vi "test - TMO of Sync-Reply.vi"(8 "error in (no error)":errorcluster, 11 "TestCase in":refnum<class "testcase-Basic-Function.lvclass">) -> (0 "error out":errorcluster, 3 "TestCase out":refnum<class "testcase-Basic-Function.lvclass">)   [LabVIEW 2017, in "testcase-Basic-Function.lvclass"]
uses:
  testcase-Basic-Function.lvclass
  src/user.lib/_NEVSTOP/Communicable State Machine(CSM)/AdvanceAPI/CSM - Revert Arguments-Safe String.vi
  src/user.lib/_NEVSTOP/Communicable State Machine(CSM)/_Shared/Trim Single-line Text.vi
  src/user.lib/_NEVSTOP/Communicable State Machine(CSM)/AdvanceAPI/CSM - Make String Arguments Safe.vi
  src/user.lib/_NEVSTOP/Communicable State Machine(CSM)/AdvanceAPI/CSM - Break Down Multiple States String.vi
  src/user.lib/_NEVSTOP/Communicable State Machine(CSM)/AdvanceAPI/CSM - Compact Multiple States.vi
  src/user.lib/_NEVSTOP/Communicable State Machine(CSM)/AdvanceAPI/CSM - Keywords.vi
  <vilib>/addons/_JKI Toolkits/VI Tester/TestCase.llb/TestCase.lvclass
  src/user.lib/_NEVSTOP/Communicable State Machine(CSM)/Communicable State Machine.lvlib
  C:/Program Files (x86)/National Instruments/LabVIEW 2017/vi.lib/addons/_JKI Toolkits/VI Tester/TestCase.llb/TestCase.lvclass
panel:
  out "x-y":u32
  out "State History":string
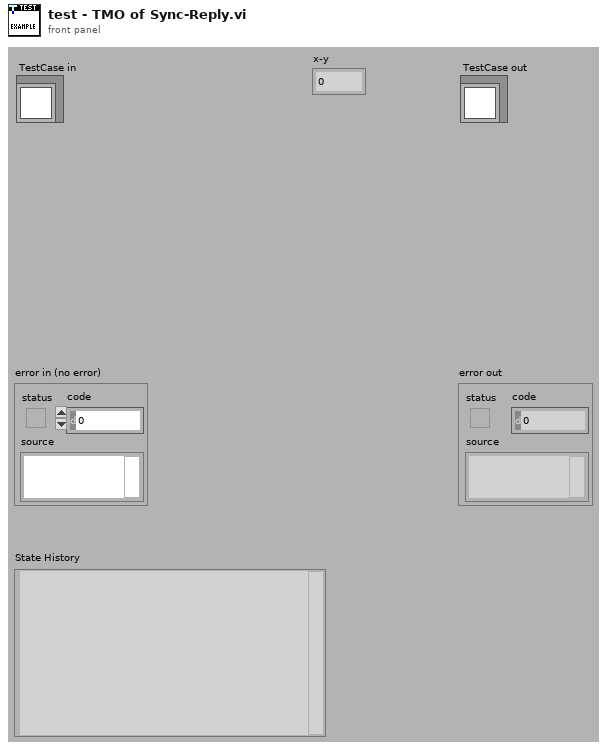
[diagram p1: front panel]
types:
  T1 = enum32{"Invalid", "Standard", "Closed", "Hidden", "Minimized", "Maximized"}
  T2 = enum32{"invalid app kind", "Development System", "Run Time System", "Student Edition", "Embedded LabVIEW", "Evaluation", "Custom"}
  T3 = typedef "Communicable State Machine.lvlib/_CSM_Response Source Message.ctl" = cluster{"‘State":string, "’Arguments":string, "’Error":errorcluster}
  T4 = cluster{"Current VI Reference":refnum<vi>, "Close Panel on Exit?":bool}
  T5 = cluster{"Core":cluster{"Current VI Reference":refnum<vi>, "Close Panel on Exit?":bool}, "Your Boolean data":bool, "Your string data":string}
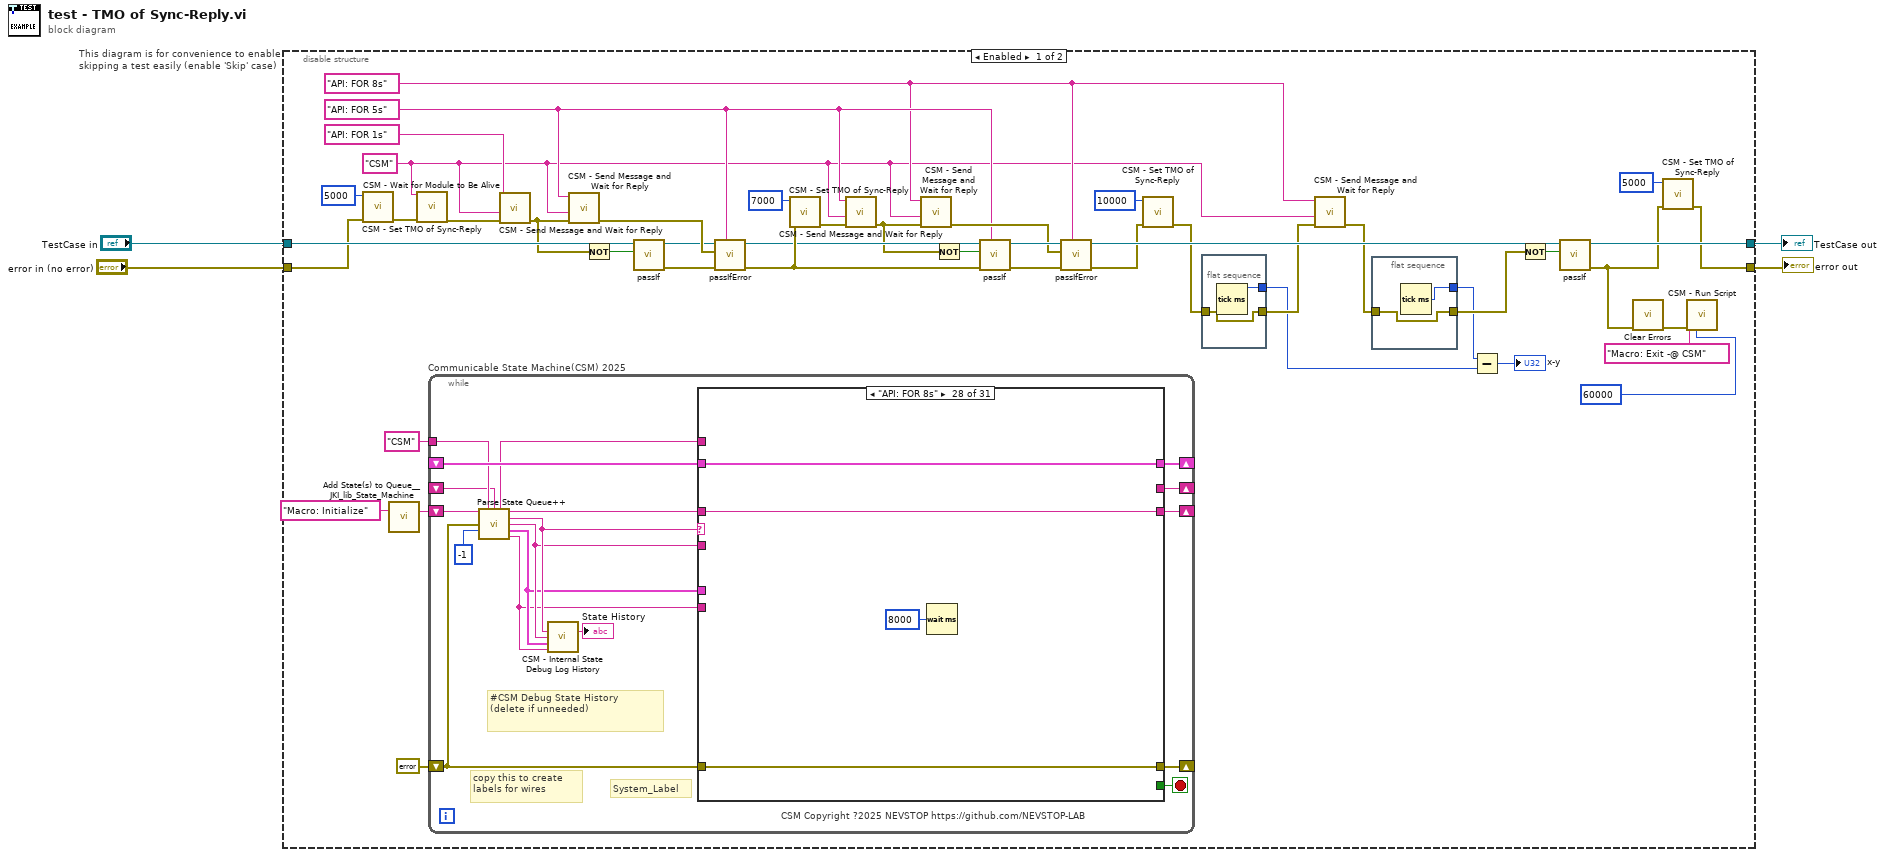
[diagram p0: block diagram]
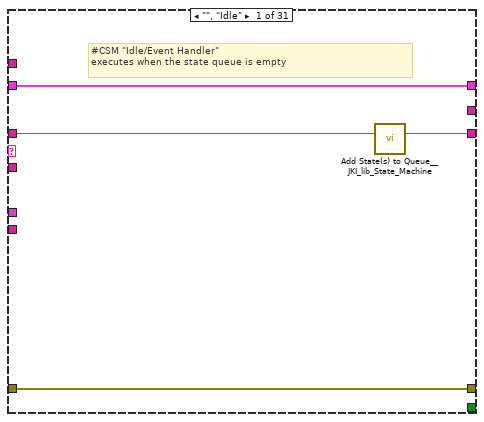
[diagram p2: hidden frame]
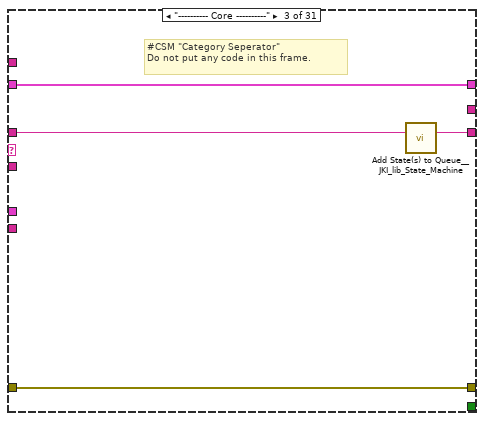
[diagram p4: hidden frame]
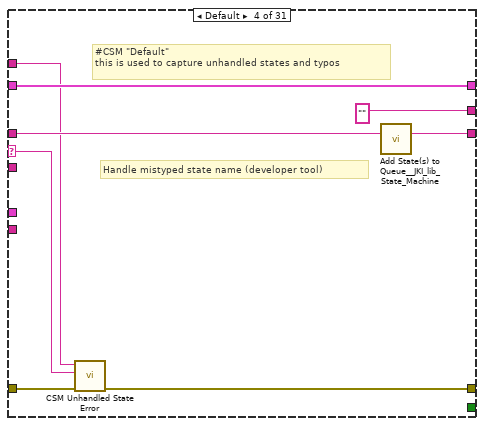
[diagram p5: hidden frame]
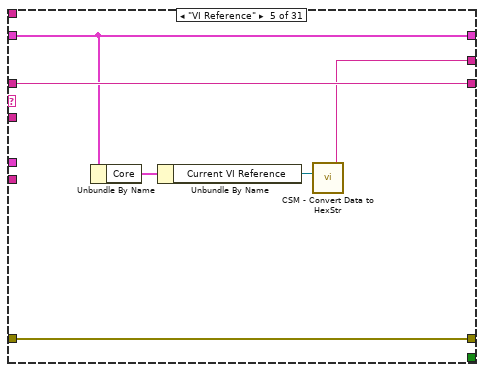
[diagram p6: hidden frame]
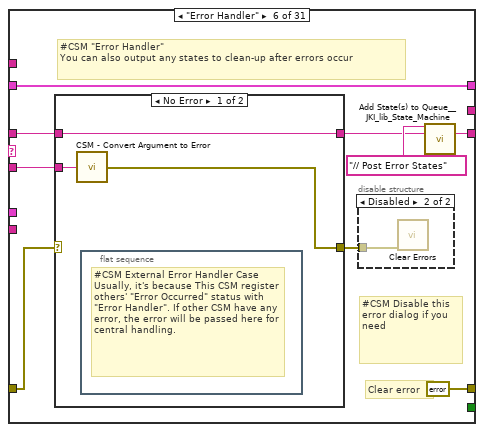
[diagram p7: hidden frame]
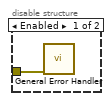
[diagram p8: hidden frame]
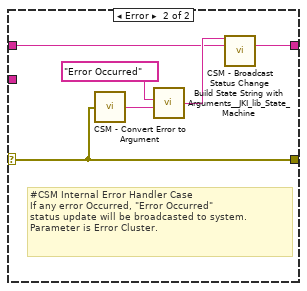
[diagram p9: hidden frame]
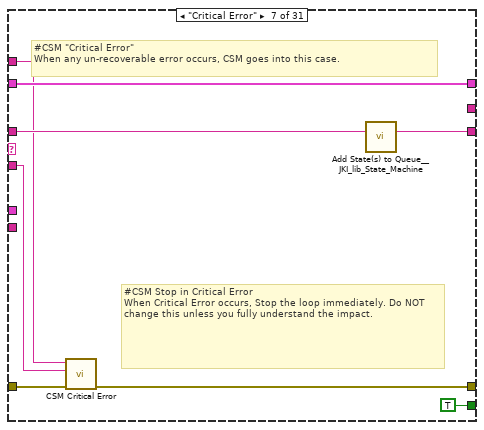
[diagram p10: hidden frame]
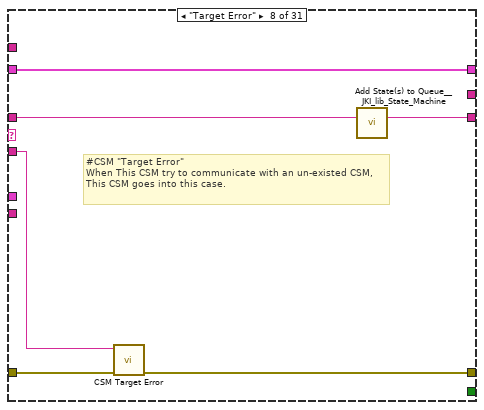
[diagram p11: hidden frame]
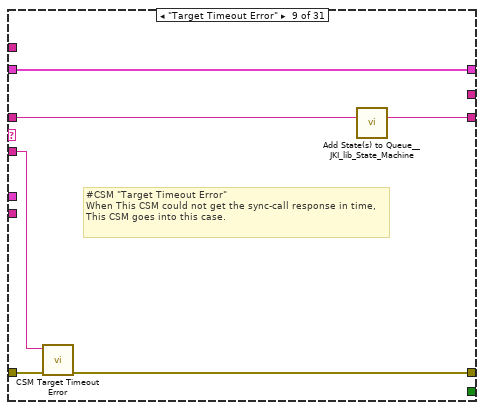
[diagram p12: hidden frame]
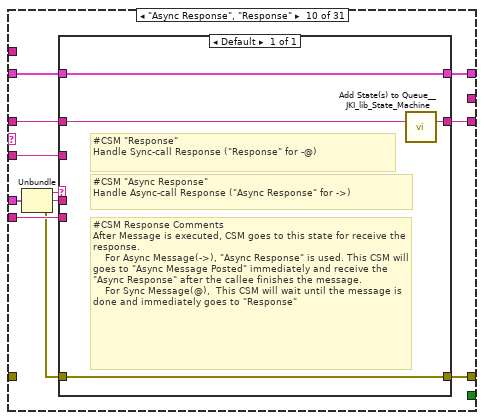
[diagram p13: hidden frame]
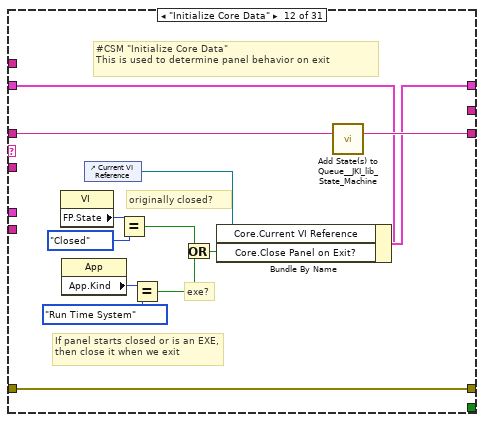
[diagram p15: hidden frame]
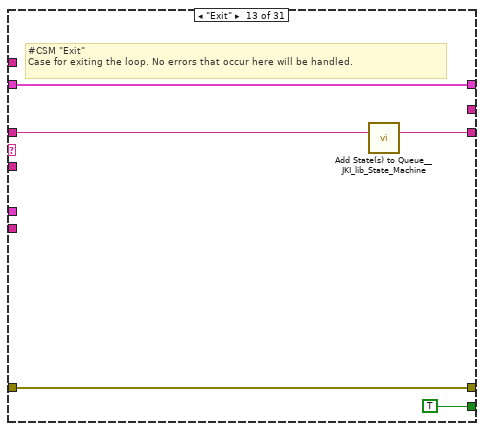
[diagram p16: hidden frame]
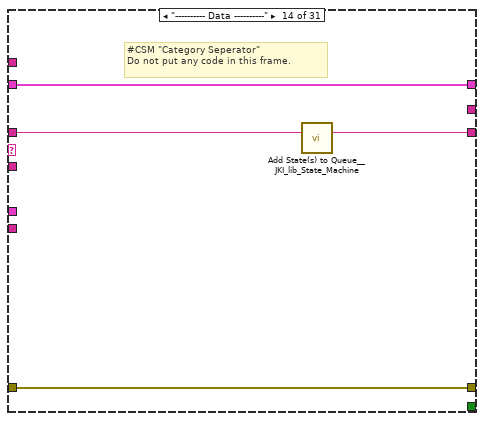
[diagram p17: hidden frame]
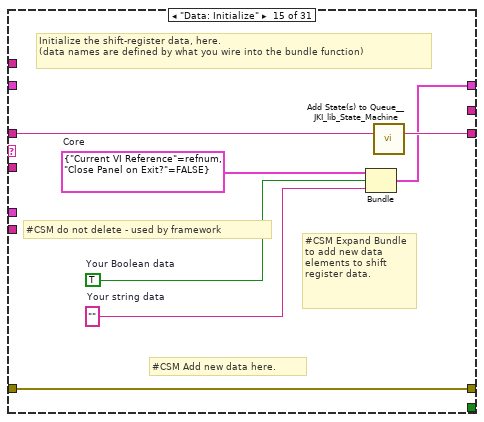
[diagram p18: hidden frame]
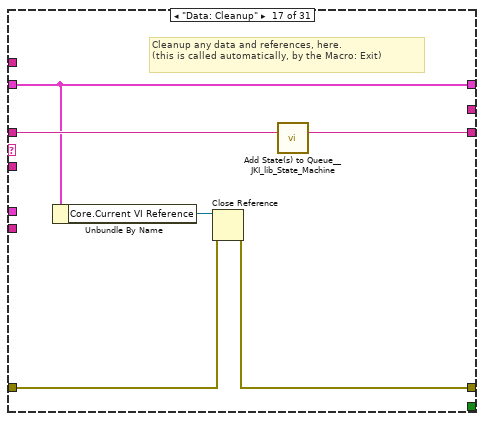
[diagram p20: hidden frame]
diagram:
  n1 = disable-structure "This diagram is for convenience to enable skipping a test easily (enable 'Skip' case)" shown="Enabled" {
    disable-tunnel: "TestCase in" -> [w41 w333]
    disable-tunnel: [w22 w331] -> w1
    disable-tunnel: [w6 w332] -> w3
    disable-tunnel: "error in (no error)" -> [w14 w330]
    frame Enabled {
      w24 = "API: FOR 8s" ("State")
      w28 = "API: FOR 5s" ("State")
      w19 = "CSM" ("Name (\"\" to Use UUID)")
      n2 = call "CSM - Set TMO of Sync-Reply.vi"("Error In"=w14, "TMO For Sync-Rep (ms) In"=5000 ("TMO for Sync-Rep(ms)")) -> ("error out"=w15:errorcluster)  [unwired: 8 in, 1 out]
      n3 = call <vilib>:"Add State(s) to Queue__JKI_lib_State_Machine.vi"("State(s) in (\"\")"="Macro: Initialize" ("Init State(\"Macro: Initialize\")")) -> ("States Out"=w49:string)  [unwired: 14 in]
      n4 = call "CSM - Wait for Module to Be Alive.vi"("CSM Name"=w19, "error in (no error)"=w15) -> ("error out"=w45:errorcluster)  [unwired: 11 in, 2 out]
      n5 = while "Communicable State Machine(CSM) 2025" {
        shift-right: [w66] -> _
        shift-left: _ -> [w65]
        shift-right: [w69] -> _
        shift-left: errorcluster {"status"=FALSE, "code"=0, "source"=""} ("error out") -> [w64]
        shift-right: [w68] -> _
        shift-left: w49 -> [w70]
        tunnel: "CSM" ("Name (\"\" to Use UUID)") -> [w62]
        shift-right: [w63] -> _
        shift-left: _ -> [w56]
        stop <- w67 stop-if-true
        # "#CSM Debug State History\n(delete if unneeded)"
        # "copy this to create labels for wires"
        # "System_Label"
        # "CSM Copyright ?2025 NEVSTOP https://github.com/NEVSTOP-LAB"
        n6 = call "Parse State Queue++.vi"("State Queue"=w70, "Name (\"\" to Use UUID)"=w62, "Response Arguments"=w56, "Previous Error"=w64, "Dequeue (1 ms)"=-1 ("Timeout")) -> ("Name Used"=w57:string, "Remaining States"=w71:string, "Current State"=w61:string, "Arguments"=w60:string, "Additional Information"=w59:T3, "Source CSM"=w58:string)  [unwired: 5 in]
        n7 = call "CSM - Internal State Debug Log History.vi"("State"=w61, "Arguments (\"\")"=w60, ">> Response Source Message >>"=w59, "Source (\"\")"=w58) -> ("Debug Log"=→"State History":string)  [unwired: 11 in]
        n8 = case shown="\"API: FOR 8s\"" w61 {
          selector: w61 -> [_ _ _ w85 _ _ _ _ _ _ _ _ _ _ _ _ _ _ _ _ _ _ _ _ _ _ _ _ _ _ _]
          tunnel: w71 -> [w72 w77 w82 w89 w95 w101 w122 w128 w134 w142 w153 w167 w172 w176 w183 w185 w192 w196 w200 w206 w221 w290 w295 w302 w304 w308 w312 w316 w321 w325 w329]
          tunnel: w60 -> [_ _ _ _ _ w100 w118 w127 w132 w141 _ _ _ _ _ _ _ _ _ w201 w215 _ _ _ _ _ _ _ _ _ _]
          tunnel: w65 -> [w73 w76 w79 w87 w94 w104 w123 w129 w135 w144 w152 w160 w170 w173 _ w184 w187 w193 w198 w204 w217 w287 w292 w299 w303 w307 w311 w315 w318 w322 w326]
          tunnel: [w74 w78 w80 w83 w96 errorcluster {"status"=FALSE, "code"=0, "source"=""} ("error out") w119 w125 w131 w147 w154 w164 w169 w174 w180 w186 w188 w194 w197 w202 w218 w288 w293 w300 w305 w309 w313 w317 w319 w323 w327] -> w69
          tunnel: w64 -> [w74 w78 w80 w90 w96 w102 w124 w126 w133 _ w154 w164 w169 w174 w180 w186 w189 w194 w197 w203 w219 w288 w293 w300 w305 w309 w313 w317 w319 w323 w327]
          tunnel: [w75 w77 w81 w88 w95 w97 w121 w130 w136 w143 w153 w166 w171 w175 w182 w185 w191 w195 w199 w205 w220 w289 w294 w301 w304 w308 w312 w316 w320 w324 w328] -> w68
          tunnel: [_ _ _ _ _ _ TRUE _ _ _ _ _ TRUE _ _ _ _ _ _ _ _ _ _ _ _ _ _ _ _ _ _] -> w67
          tunnel: [w73 w76 w79 w87 w94 w104 w123 w129 w135 w145 w152 w165 w170 w173 w181 w184 w187 w193 w198 w204 w217 w287 w292 w299 w303 w307 w311 w315 w318 w322 w326] -> w66
          tunnel: w58 -> [_ _ _ _ _ _ _ _ _ w139 _ _ _ _ _ _ _ _ _ _ _ _ _ _ _ _ _ _ _ _ _]
          tunnel: w59 -> [_ _ _ _ _ _ _ _ _ w146 _ _ _ _ _ _ _ _ _ _ _ _ _ _ _ _ _ _ _ _ _]
          tunnel: [_ _ _ "" w91 _ _ _ _ _ _ _ _ _ _ _ _ _ _ _ _ _ _ _ _ _ _ _ _ _ _] -> w63
          tunnel: w57 -> [_ _ _ w84 _ _ w117 _ _ _ _ _ _ _ _ _ _ _ _ _ _ _ _ _ _ _ _ _ _ _ _]
          frame "", "Idle" {
            # "#CSM \"Idle/Event Handler\"\nexecutes when the state queue is empty"
            n9 = call <vilib>:"Add State(s) to Queue__JKI_lib_State_Machine.vi"("State(s) in (\"\")"=w72) -> ("States Out"=w75:string)  [unwired: 14 in]
          }
          frame "CSM Documentation" {
            # "#CSM README FIRST\n\nCommunicable State Machine(CSM) is a LabVIEW application framework that builds upon JKI State Machine(JKISM). It follows the pattern of JKISM and extends the keywords to describe message communication between modules, including concepts such as Sync-Message, Async-Message, Subscription/Unsubscription of status - essential elements for creating reusable code modules. For more information, please visit the CSM wiki: https://nevstop-lab.github.io/CSM-Wiki/\n\nFor instructions on JKI State Machine, visit: http://jki.net/state-machine/\nFor information about CSM, visit: https://github.com/NEVSTOP-LAB"
            # "#CSM \"Documentation\"\nCase for holding CSM Documenation"
          }
          frame "---------- Core ----------" {
            # "#CSM \"Category Seperator\"\nDo not put any code in this frame."
            n10 = call <vilib>:"Add State(s) to Queue__JKI_lib_State_Machine.vi"("State(s) in (\"\")"=w82) -> ("States Out"=w81:string)  [unwired: 14 in]
          }
          frame Default {
            # "#CSM \"Default\"\nthis is used to capture unhandled states and typos"
            # "Handle mistyped state name (developer tool)"
            n11 = call "CSM Unhandled State Error.vi"("error in (no error)"=w90, "Undefined State"=w85, "CSM Name"=w84) -> ("error out"=w83:errorcluster)  [unwired: 8 in]
            n12 = call <vilib>:"Add State(s) to Queue__JKI_lib_State_Machine.vi"("State(s) in (\"\")"=w89) -> ("States Out"=w88:string)  [unwired: 14 in]
          }
          frame "VI Reference" {
            n13 = Unbundle By Name(w94) -> ("Core"=w93:T4)
            n14 = Unbundle By Name(w93) -> ("Current VI Reference"=w92:refnum<vi>)
            n15 = call "CSM - Convert Data to HexStr.vi"("Variant"=w92) -> ("HEX String (0-9,A-F)"=w91:string)  [unwired: 8 in]
          }
          frame "Error Handler" {
            # "#CSM Disable this error dialog if you need"
            # "#CSM \"Error Handler\"\nYou can also output any states to clean-up after errors occur"
            # "Clear error"
            n16 = case shown="No Error" w102 {
              selector: w102 -> [_ w111]
              tunnel: [w110 w113] -> w98
              tunnel: w101 -> [w110 w112]
              tunnel: w100 -> [w109 _]
              tunnel: [w108 w111] -> w103
              frame No Error {
                n17 = call "CSM - Convert Argument to Error.vi"("Argument"=w109) -> ("Error"=w108:errorcluster)  [unwired: 4 in]
                n18 = flat-sequence {
                  frame #0 {
                    # "#CSM External Error Handler Case\nUsually, it's because This CSM register others' \"Error Occurred\" status with \"Error Handler\". If other CSM have any error, the error will be passed here for central handling."
                  }
                }
              }
              frame Error {
                # "#CSM Internal Error Handler Case \nIf any error Occurred, \"Error Occurred\" \nstatus update will be broadcasted to system.\nParameter is Error Cluster."
                n19 = call "CSM - Convert Error to Argument.vi"("Error"=w111) -> ("Argument"=w115:string)  [unwired: 4 in]
                n20 = call <vilib>:"Build State String with Arguments__JKI_lib_State_Machine.vi"("Arguments (\"\")"=w115, "State"="Error Occurred" ("Status with Arguments")) -> ("State with Arguments"=w114:string)  [unwired: 4 in]
                n21 = call "CSM - Broadcast Status Change.vi"("Status With Arguments"=w114, "State Queue"=w112) -> ("Remaining States"=w113:string)  [unwired: 13 in]
              }
            }
            n22 = disable-structure shown="Disabled" {
              disable-tunnel: w103 -> [w106 w107]
              frame Enabled {
                n23 = call <vilib>:"General Error Handler.vi"("error in (no error)"=w106) -> ()  [unwired: 10 in, 5 out]
              }
              frame Disabled {
                n24 = call <vilib>:"Clear Errors.vi"("error in (no error)"=w107) -> ()  [unwired: 5 in, 2 out]
              }
            }
            n25 = call <vilib>:"Add State(s) to Queue__JKI_lib_State_Machine.vi"("State(s) in Front (\"\")"="// Post Error States", "State(s) in (\"\")"=w98) -> ("States Out"=w97:string)  [unwired: 13 in]
          }
          frame "Critical Error" {
            # "#CSM Stop in Critical Error\nWhen Critical Error occurs, Stop the loop immediately. Do NOT change this unless you fully understand the impact."
            # "#CSM \"Critical Error\"\nWhen any un-recoverable error occurs, CSM goes into this case."
            n26 = call "CSM Critical Error.vi"("error in (no error)"=w124, "Arugments (As Reason)"=w118, "CSM Name"=w117) -> ("error out"=w119:errorcluster)  [unwired: 8 in]
            n27 = call <vilib>:"Add State(s) to Queue__JKI_lib_State_Machine.vi"("State(s) in (\"\")"=w122) -> ("States Out"=w121:string)  [unwired: 14 in]
          }
          frame "Target Error" {
            # "#CSM \"Target Error\"\nWhen This CSM try to communicate with an un-existed CSM, This CSM goes into this case."
            n28 = call "CSM Target Error.vi"("error in (no error)"=w126, "Arguments (As CSM Name)"=w127) -> ("error out"=w125:errorcluster)  [unwired: 9 in]
            n29 = call <vilib>:"Add State(s) to Queue__JKI_lib_State_Machine.vi"("State(s) in (\"\")"=w128) -> ("States Out"=w130:string)  [unwired: 14 in]
          }
          frame "Target Timeout Error" {
            # "#CSM \"Target Timeout Error\"\nWhen This CSM could not get the sync-call response in time, This CSM goes into this case."
            n30 = call "CSM Target Timeout Error.vi"("error in (no error)"=w133, "Arguments (As CSM Name)"=w132) -> ("error out"=w131:errorcluster)  [unwired: 9 in]
            n31 = call <vilib>:"Add State(s) to Queue__JKI_lib_State_Machine.vi"("State(s) in (\"\")"=w134) -> ("States Out"=w136:string)  [unwired: 14 in]
          }
          frame "Async Response", "Response" {
            n32 = Unbundle(w146) -> ("‘State"=w140:string, "’Arguments"=w138:string, "’Error"=w137:errorcluster)
            n33 = case shown="Default" w140 {
              tunnel: [w151] -> w147
              tunnel: w137 -> [w151]
              tunnel: [w150] -> w145
              tunnel: w144 -> [w150]
              tunnel: [w148] -> w143
              tunnel: w142 -> [w149]
              tunnel: w141 -> [_]
              tunnel: w139 -> [_]
              tunnel: w138 -> [_]
              frame Default {
                # "#CSM Response Comments\nAfter Message is executed, CSM goes to this state for receive the response.\n    For Async Message(->), \"Async Response\" is used. This CSM will goes to \"Async Message Posted\" immediately and receive the \"Async Response\" after the callee finishes the message.\n    For Sync Message(@),  This CSM will wait until the message is done and immediately goes to \"Response\""
                # "#CSM \"Async Response\"\nHandle Async-call Response (\"Async Response\" for ->)"
                # "#CSM \"Response\"\nHandle Sync-call Response (\"Response\" for -@)"
                n34 = call <vilib>:"Add State(s) to Queue__JKI_lib_State_Machine.vi"("State(s) in (\"\")"=w149) -> ("States Out"=w148:string)  [unwired: 14 in]
              }
            }
          }
          frame "Async Message Posted" {
            # "#CSM \"Async Message Posted\"\nAfter Async Message is posted (-> or ->| ), CSM goes to this state for post-action.\nYou can use Argument - State to tell which Async Message is called."
          }
          frame "Initialize Core Data" {
            # "#CSM \"Initialize Core Data\"\nThis is used to determine panel behavior on exit"
            # "originally closed?"
            # "exe?"
            # "If panel starts closed or is an EXE, then close it when we exit"
            n35 = property class="VI"() -> ("FP.State"=w157:T1)  [unwired: 2 in, 2 out]
            n36 = property class="App"() -> ("App.Kind"=w163:T2)  [unwired: 2 in, 2 out]
            n37 = control-ref of="Current VI Reference"() -> (w158:refnum<vi>)
            n38 = Equal?(x=w157, y=T1."Closed" ("Front Panel Window:State")) -> (x = y?=w155:bool)
            n39 = Equal?(x=w163, y=T2."Run Time System" ("Application:Kind")) -> (x = y?=w161:bool)
            n40 = Or(x=w155, y=w161) -> (x .or. y?=w159:bool)
            n41 = Bundle By Name(cluster=w160, "Core.Current VI Reference"=w158, "Core.Close Panel on Exit?"=w159) -> (w165:T5)
            n42 = call <vilib>:"Add State(s) to Queue__JKI_lib_State_Machine.vi"("State(s) in (\"\")"=w167) -> ("States Out"=w166:string)  [unwired: 14 in]
          }
          frame "Exit" {
            # "#CSM \"Exit\"\nCase for exiting the loop. No errors that occur here will be handled."
            n43 = call <vilib>:"Add State(s) to Queue__JKI_lib_State_Machine.vi"("State(s) in (\"\")"=w172) -> ("States Out"=w171:string)  [unwired: 14 in]
          }
          frame "---------- Data ----------" {
            # "#CSM \"Category Seperator\"\nDo not put any code in this frame."
            n44 = call <vilib>:"Add State(s) to Queue__JKI_lib_State_Machine.vi"("State(s) in (\"\")"=w176) -> ("States Out"=w175:string)  [unwired: 14 in]
          }
          frame "Data: Initialize" {
            w177 = T4 {"Current VI Reference"=refnum, "Close Panel on Exit?"=FALSE}  # Core
            w179 = TRUE  # Your Boolean data
            w178 = ""  # Your string data
            # "#CSM do not delete - used by framework"
            # "#CSM Expand Bundle to add new data elements to shift register data."
            # "#CSM Add new data here."
            # "Initialize the shift-register data, here.\n(data names are defined by what you wire into the bundle function)"
            n45 = Bundle("Core"=w177, "Your Boolean data"=w179, "Your string data"=w178) -> (w181:T5)  [unwired: 1 in]
            n46 = call <vilib>:"Add State(s) to Queue__JKI_lib_State_Machine.vi"("State(s) in (\"\")"=w183) -> ("States Out"=w182:string)  [unwired: 14 in]
          }
          frame "Data: Update Indicators" {
          }
          frame "Data: Cleanup" {
            # "Cleanup any data and references, here.\n(this is called automatically, by the Macro: Exit)"
            n47 = Unbundle By Name(w187) -> ("Core.Current VI Reference"=w190:refnum<vi>)
            n48 = Close Reference(reference=w190, error in (no error)=w189) -> (error out=w188:errorcluster)
            n49 = call <vilib>:"Add State(s) to Queue__JKI_lib_State_Machine.vi"("State(s) in (\"\")"=w192) -> ("States Out"=w191:string)  [unwired: 14 in]
          }
          frame "---------- UI ----------" {
            # "#CSM \"Category Seperator\"\nDo not put any code in this frame."
            n50 = call <vilib>:"Add State(s) to Queue__JKI_lib_State_Machine.vi"("State(s) in (\"\")"=w196) -> ("States Out"=w195:string)  [unwired: 14 in]
          }
          frame "UI: Initialize" {
            # "#CSM \"UI: Initialize\"\nInitialize the User Interface, here.\n(this is called automatically, by the Macro: Init)"
            n51 = call <vilib>:"Add State(s) to Queue__JKI_lib_State_Machine.vi"("State(s) in (\"\")"=w200) -> ("States Out"=w199:string)  [unwired: 14 in]
          }
          frame "UI: Cursor Set" {
            # "#CSM \"UI: Cursor Set\"\nSet and Unset Cursor Busy.\n(Usage: \"UI: Cursor Set >> Busy|Idle\")"
            # "Argument"
            n52 = disable-structure shown="TARGET_TYPE!=Windows" {
              disable-tunnel: w203 -> [w209 w214]
              disable-tunnel: [w208 w214] -> w202
              disable-tunnel: w201 -> [w207 _]
              frame condition #0 (active) {
                n53 = case shown="\"Idle\", Default" w207 {
                  tunnel: w209 -> [w211 w213]
                  tunnel: [w210 w212] -> w208
                  frame "Idle", Default {
                    n54 = call <vilib>:"Unset Busy.vi"("error in (no error)"=w211) -> ("error out"=w210:errorcluster)  [unwired: 10 in]
                  }
                  frame "Busy" {
                    n55 = call <vilib>:"Set Busy.vi"("error in (no error)"=w213) -> ("error out"=w212:errorcluster)  [unwired: 9 in, 1 out]
                  }
                }
              }
              frame condition #1 {
              }
            }
            n56 = call <vilib>:"Add State(s) to Queue__JKI_lib_State_Machine.vi"("State(s) in (\"\")"=w206) -> ("States Out"=w205:string)  [unwired: 14 in]
          }
          frame "UI: Front Panel State" {
            # "#CSM \"UI: Front Panel State\"\nSet Front Panel Open or Closed\n(Usage: \"UI: Front Panel State >> Open|Close\")"
            # "Argument"
            n57 = Unbundle By Name(w217) -> ("Core.Current VI Reference"=w216:refnum<vi>)
            n58 = call <vilib>:"Add State(s) to Queue__JKI_lib_State_Machine.vi"("State(s) in (\"\")"=w221) -> ("States Out"=w220:string)  [unwired: 14 in]
            n59 = case shown="\"Close\", \"Closed\"" w215 {
              tunnel: w219 -> [w227 w242 w253 w266 w279]
              tunnel: [w229 w243 w255 w268 w281] -> w218
              tunnel: w216 -> [w228 w240 w254 w267 w280]
              frame "Open", "Standard", Default {
                w222 = T1."Standard" ("State")
                n60 = property class="VI"(reference=w228, error in=w227) -> (reference out=w225:refnum<vi>, error out=w226:errorcluster, "FP.State"=w224:T1)
                n61 = Not Equal?(x=w224, y=w222) -> (x != y?=w223:bool)
                n62 = case shown="True" w223 {
                  tunnel: [w233 w235] -> w229
                  tunnel: w226 -> [w232 w235]
                  tunnel: w225 -> [w231 _]
                  tunnel: w222 -> [w230 _]
                  frame True {
                    n63 = invoke class="VI" method="FP.Open"(reference=w231, error in=w232, "Activate"=TRUE, "State"=w230) -> (error out=w233:errorcluster)  [unwired: 1 in, 4 out]
                  }
                  frame False {
                  }
                }
              }
              frame "Close", "Closed" {
                n64 = property class="VI"(reference=w240, error in=w242) -> (reference out=w239:refnum<vi>, error out=w241:errorcluster, "FP.State"=w237:T1)
                n65 = Not Equal?(x=w237, y=T1."Closed" ("Front Panel Window:State")) -> (x != y?=w236:bool)
                n66 = case shown="False" w236 {
                  tunnel: [w244 w247] -> w243
                  tunnel: w241 -> [w244 w246]
                  tunnel: w239 -> [_ w245]
                  frame False {
                  }
                  frame True {
                    n67 = invoke class="VI" method="FP.Close"(reference=w245, error in=w246) -> (error out=w247:errorcluster)  [unwired: 1 in, 2 out]
                  }
                }
              }
              frame "Hidden", "Hide" {
                w248 = T1."Hidden" ("State")
                n68 = property class="VI"(reference=w254, error in=w253) -> (reference out=w251:refnum<vi>, error out=w252:errorcluster, "FP.State"=w250:T1)
                n69 = Not Equal?(x=w250, y=w248) -> (x != y?=w249:bool)
                n70 = case shown="True" w249 {
                  tunnel: [w259 w260] -> w255
                  tunnel: w252 -> [w258 w260]
                  tunnel: w251 -> [w257 _]
                  tunnel: w248 -> [w256 _]
                  frame True {
                    n71 = invoke class="VI" method="FP.Open"(reference=w257, error in=w258, "State"=w256) -> (error out=w259:errorcluster)  [unwired: 2 in, 4 out]
                  }
                  frame False {
                  }
                }
              }
              frame "Minimize", "Minimized" {
                w261 = T1."Minimized" ("State")
                n72 = property class="VI"(reference=w267, error in=w266) -> (reference out=w264:refnum<vi>, error out=w265:errorcluster, "FP.State"=w263:T1)
                n73 = Not Equal?(x=w263, y=w261) -> (x != y?=w262:bool)
                n74 = case shown="True" w262 {
                  tunnel: [w272 w273] -> w268
                  tunnel: w265 -> [w271 w273]
                  tunnel: w264 -> [w270 _]
                  tunnel: w261 -> [w269 _]
                  frame True {
                    n75 = invoke class="VI" method="FP.Open"(reference=w270, error in=w271, "State"=w269) -> (error out=w272:errorcluster)  [unwired: 2 in, 4 out]
                  }
                  frame False {
                  }
                }
              }
              frame "Maximize", "Maximized" {
                w274 = T1."Maximized" ("State")
                n76 = property class="VI"(reference=w280, error in=w279) -> (reference out=w277:refnum<vi>, error out=w278:errorcluster, "FP.State"=w276:T1)
                n77 = Not Equal?(x=w276, y=w274) -> (x != y?=w275:bool)
                n78 = case shown="True" w275 {
                  tunnel: [w285 w286] -> w281
                  tunnel: w278 -> [w284 w286]
                  tunnel: w277 -> [w283 _]
                  tunnel: w274 -> [w282 _]
                  frame True {
                    n79 = invoke class="VI" method="FP.Open"(reference=w283, error in=w284, "State"=w282) -> (error out=w285:errorcluster)  [unwired: 2 in, 4 out]
                  }
                  frame False {
                  }
                }
              }
            }
          }
          frame "---------- Macro ----------" {
            # "#CSM \"Category Seperator\"\nDo not put any code in this frame."
            n80 = call <vilib>:"Add State(s) to Queue__JKI_lib_State_Machine.vi"("State(s) in (\"\")"=w290) -> ("States Out"=w289:string)  [unwired: 14 in]
          }
          frame "Macro: Initialize" {
            # "#CSM \"Macro: Initialize\"\nInitialization Macro (This is called once, when the VI starts)"
            n81 = call <vilib>:"Add State(s) to Queue__JKI_lib_State_Machine.vi"("State(s) in Front (\"\")"="Data: Initialize\nInitialize Core Data\nData: Update Indicators", "State(s) in (\"\")"=w295) -> ("States Out"=w294:string)  [unwired: 13 in]
          }
          frame "Macro: Exit" {
            # "#CSM \"Macro: Exit\"\nExit Macro (This is called once, when the VI exits)"
            n82 = call <vilib>:"Add State(s) to Queue__JKI_lib_State_Machine.vi"("State(s) in Front (\"\")"="//Exit Sub-Modules ", "State(s) at Back (\"\")"="Data: Cleanup\nExit") -> ("States Out"=w297:string)  [unwired: 13 in]
            n83 = call <vilib>:"Add State(s) to Queue__JKI_lib_State_Machine.vi"("State(s) in Front (\"\")"=w297, "State(s) in (\"\")"=w302) -> ("States Out"=w301:string)  [unwired: 13 in]
          }
          frame "---------- API ----------" {
            # "#CSM \"Category Seperator\"\nDo not put any code in this frame."
          }
          frame "API: FOR 5s" {
            n84 = Wait (ms)(milliseconds to wait=u32 5000) -> ()  [unwired: 1 out]
          }
          frame "API: FOR 1s" {
            n85 = Wait (ms)(milliseconds to wait=u32 1000) -> ()  [unwired: 1 out]
          }
          frame "API: FOR 8s" {
            n86 = Wait (ms)(milliseconds to wait=u32 8000) -> ()  [unwired: 1 out]
          }
          frame "---------- Action ----------" {
            # "#CSM \"Category Seperator\"\nDo not put any code in this frame."
            n87 = call <vilib>:"Add State(s) to Queue__JKI_lib_State_Machine.vi"("State(s) in (\"\")"=w321) -> ("States Out"=w320:string)  [unwired: 14 in]
          }
          frame "Action: action1" {
            # "#CSM \"Internal State\"\nThis category is used for holding internal states"
            n88 = call <vilib>:"Add State(s) to Queue__JKI_lib_State_Machine.vi"("State(s) in (\"\")"=w325) -> ("States Out"=w324:string)  [unwired: 14 in]
          }
          frame "Action: action2" {
            # "#CSM \"Internal State\"\nThis category is used for holding internal states"
            n89 = call <vilib>:"Add State(s) to Queue__JKI_lib_State_Machine.vi"("State(s) in (\"\")"=w329) -> ("States Out"=w328:string)  [unwired: 14 in]
          }
        }
      }
      n90 = call "CSM - Send Message and Wait for Reply.vi"("Error In (No Error)"=w45, "Target Module"=w19, "State"="API: FOR 1s") -> ("error out"=w17:errorcluster)  [unwired: 6 in, 2 out]
      n91 = call "CSM - Send Message and Wait for Reply.vi"("Error In (No Error)"=w17, "Target Module"=w19, "State"=w28) -> ("error out"=w43:errorcluster)  [unwired: 6 in, 2 out]
      n92 = Not(x=w17) -> (.not. x?=w42:bool)
      n93 = call-dynamic "passIf.vi"("pass"=w42, "TestCase in"=w41) -> ("error out"=w39:errorcluster, "TestCase out"=w40:refnum<class "testcase-Basic-Function.lvclass">)  [unwired: 8 in]
      n94 = call-dynamic "passIfError.vi"("custom report message (\"\")"=w28, "error in (no error)"=w39, "error"=w43, "TestCase in"=w40) -> ("error out"=w32:errorcluster, "TestCase out"=w31:refnum<class "testcase-Basic-Function.lvclass">)  [unwired: 6 in]
      n95 = call "CSM - Set TMO of Sync-Reply.vi"("Error In"=w32, "TMO For Sync-Rep (ms) In"=7000 ("TMO for Sync-Rep(ms)")) -> ("error out"=w33:errorcluster)  [unwired: 8 in, 1 out]
      n96 = call "CSM - Send Message and Wait for Reply.vi"("Error In (No Error)"=w33, "Target Module"=w19, "State"=w28) -> ("error out"=w18:errorcluster)  [unwired: 6 in, 2 out]
      n97 = call "CSM - Send Message and Wait for Reply.vi"("Error In (No Error)"=w18, "Target Module"=w19, "State"=w24) -> ("error out"=w34:errorcluster)  [unwired: 6 in, 2 out]
      n98 = Not(x=w18) -> (.not. x?=w35:bool)
      n99 = call-dynamic "passIf.vi"("custom report message (\"\")"=w28, "error in (no error)"=w32, "pass"=w35, "TestCase in"=w31) -> ("error out"=w37:errorcluster, "TestCase out"=w36:refnum<class "testcase-Basic-Function.lvclass">)  [unwired: 6 in]
      n100 = call-dynamic "passIfError.vi"("custom report message (\"\")"=w24, "error in (no error)"=w37, "error"=w34, "TestCase in"=w36) -> ("error out"=w26:errorcluster, "TestCase out"=w27:refnum<class "testcase-Basic-Function.lvclass">)  [unwired: 6 in]
      n101 = call "CSM - Set TMO of Sync-Reply.vi"("Error In"=w26, "TMO For Sync-Rep (ms) In"=10000 ("TMO for Sync-Rep(ms)")) -> ("error out"=w25:errorcluster)  [unwired: 8 in, 1 out]
      n102 = flat-sequence {
        tunnel: w25 -> [w52]
        tunnel: [w52] -> w13
        tunnel: [w53] -> w10
        frame #0 {
          n103 = Tick Count (ms)() -> (millisecond timer value=w53:u32)
        }
      }
      n104 = call "CSM - Send Message and Wait for Reply.vi"("Error In (No Error)"=w13, "Target Module"=w19, "State"=w24) -> ("error out"=w23:errorcluster)  [unwired: 6 in, 2 out]
      n105 = flat-sequence {
        tunnel: w23 -> [w50]
        tunnel: [w50] -> w12
        tunnel: [w51] -> w11
        frame #0 {
          n106 = Tick Count (ms)() -> (millisecond timer value=w51:u32)
        }
      }
      n107 = Subtract(x=w11, y=w10) -> (x-y=→"x-y":u32)
      n108 = Not(x=w12) -> (.not. x?=w29:bool)
      n109 = call-dynamic "passIf.vi"("pass"=w29, "TestCase in"=w27) -> ("error out"=w7:errorcluster, "TestCase out"=w22:refnum<class "testcase-Basic-Function.lvclass">)  [unwired: 8 in]
      n110 = call <vilib>:"Clear Errors.vi"("error in (no error)"=w7) -> ("error out"=w21:errorcluster)  [unwired: 5 in, 1 out]
      n111 = call "CSM - Set TMO of Sync-Reply.vi"("Error In"=w7, "TMO For Sync-Rep (ms) In"=5000 ("TMO for Sync-Rep(ms) In")) -> ("error out"=w6:errorcluster)  [unwired: 8 in, 1 out]
      n112 = call "CSM - Run Script.vi"("CSM Scripts"="Macro: Exit -@ CSM", "error in (no error)"=w21, "Response Timeout (-2 Using Global Settings)"=60000) -> ()  [unwired: 10 in, 3 out]
    }
    frame Disabled {
      # "skip test result while test is under development"
      n113 = call <vilib>:"skip.vi"("error in (no error)"=w330, "TestCase in"=w333) -> ("error out"=w332:errorcluster, "TestCase out"=w331:refnum<class "testcase-Basic-Function.lvclass">)  [unwired: 8 in]
    }
  }
  "error out" <- w3
  "TestCase out" <- w1
